vi "CheckValidReference.vi"(8 "error in":errorcluster, 11 "message ref in":refnum<class "CLM_LocalMessage_UserEvent.lvclass">) -> (0 "error out":errorcluster, 2 "valid?":bool, 3 "message ref out":refnum<class "CLM_LocalMessage_UserEvent.lvclass">)   [LabVIEW 2013, in "CLM_LocalMessage_UserEvent.lvclass"]
uses:
  CLM_LocalMessage_UserEvent.lvclass
  CLM_LocalMessage_UserEvent.lvclass/CLM_LocalMessage_UserEvent.ctl
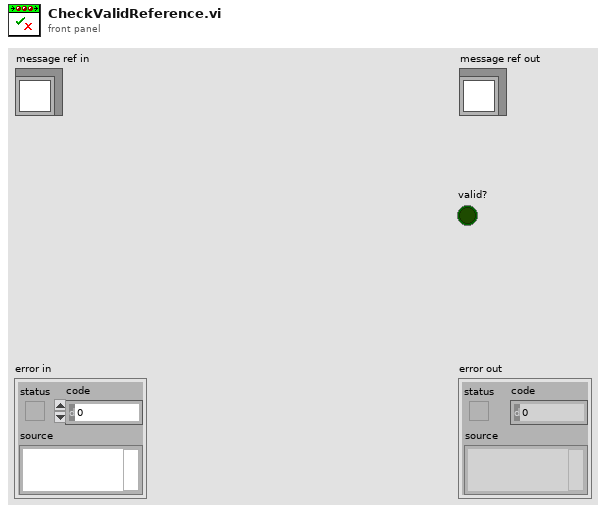
[diagram p1: front panel]
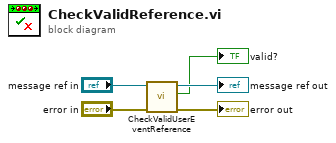
[diagram p0: block diagram]
diagram:
  n1 = call "CheckValidUserEventReference.vi"("error in"="error in", "message ref in"="message ref in") -> ("error out"=→"error out":errorcluster, "valid?"=→"valid?":bool, "message ref out"=→"message ref out":refnum<class "CLM_LocalMessage_UserEvent.lvclass">)  [unwired: 7 in]
